vi "rs3 delete context.vi"(8 "error in (no error)":errorcluster, 11 "context":u64) -> (0 "error out":errorcluster, 3 "error":u64)   [LabVIEW 2019, in "libRealSense3.lvlib"]
doc: "The final command should be to delete the CONTEXT, after all sensors, and devices have been stopped and deleted."
uses:
  libRealSense3.lvlib
  realsense2.dll
panel:
  # "RS3 Delete Context"
  # "(C) Intel Corp. 2017,  AGJ"
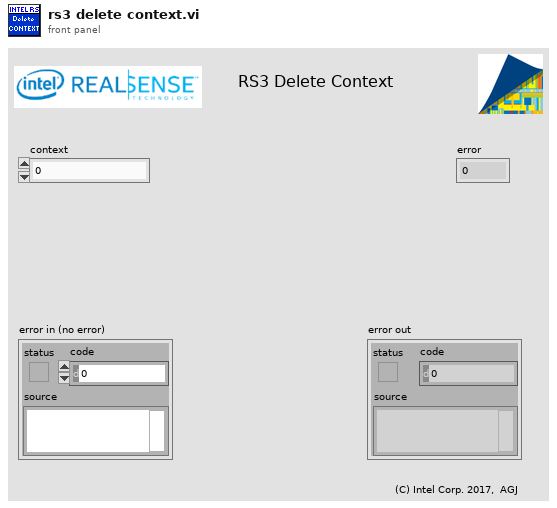
[diagram p1: front panel]
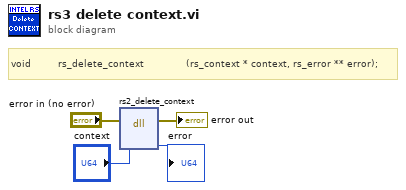
[diagram p0: block diagram]
diagram:
  # "void         rs_delete_context              (rs_context * context, rs_error ** error);"
  n1 = dll-call lib="C:/SmartekVision/Projects/RS-D4-ETH/Software/RS-SDK/wrappers/labview/realsense2.dll" fn="rs2_delete_context"(error in="error in (no error)", "context"="context") -> (error out=→"error out":errorcluster, "error"=→"error":u64)  [unwired: 5 in, 1 out]
